vi "Cheksum.vi"(8 "error in (no error)":errorcluster, 11 "Trama IN":string) -> (0 "error out":errorcluster, 3 "Trama RTS":string)   [LabVIEW 2014, in "CAP-USB.lvlib"]
doc: "Agrega el Checksum correspondiente a la trama de \nentrada al final de esa trama"
uses:
  CAP-USB.lvlib
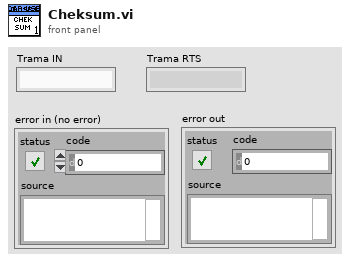
[diagram p1: front panel]
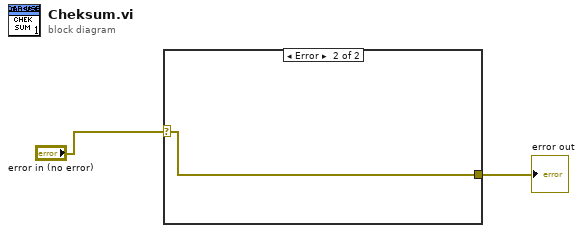
[diagram p0: block diagram]
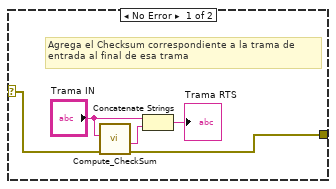
[diagram p2: hidden frame]
diagram:
  n1 = case shown="Error" "error in (no error)" {
    selector: "error in (no error)" -> [w4 w8]
    tunnel: [w3 w8] -> w1
    frame No Error {
      # "Agrega el Checksum correspondiente a la trama de \nentrada al final de esa trama"
      n2 = call "Compute_CheckSum.vi"("error in (no error)"=w4, "Trama IN"="Trama IN") -> ("error out"=w3:errorcluster, "Checksum ASCII"=w5:string)  [unwired: 8 in]
      n3 = Concatenate Strings("Trama IN", w5) -> (→"Trama RTS":string)
    }
    frame Error {
    }
  }
  "error out" <- w1
